vi "sub_ekf_jacob-f.vi"(10 "ud":T1, 11 "xEst":T1) -> (3 "jF":T1)   [LabVIEW 2019]
uses:
  <vilib>/Analysis/Matrix/Datatypes/RealMatrix.ctl
  Ctrl/cmd_common.ctl
  <vilib>/Analysis/Matrix/NI_Matrix.lvlib
panel:
  # "Jacobian of Motion Model\n\n    motion model\n    x_{t+1} = x_t+v*dt*cos(yaw)\n    y_{t+1} = y_t+v*dt*sin(yaw)\n    yaw_{t+1} = yaw_t+omega*dt\n    v_{t+1} = v{t}\n    so\n    dx/dyaw = -v*dt*sin(yaw)\n    dx/dv = dt*cos(yaw)\n    dy/dyaw = v*dt*cos(yaw)\n    dy/dv = dt*sin(yaw)\n    \"\"\""
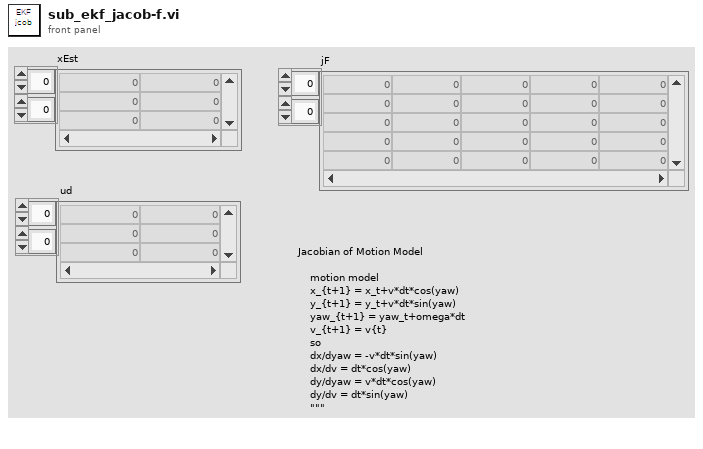
[diagram p1: front panel]
types:
  T1 = typedef "NI_Matrix.lvlib/RealMatrix.ctl" = dbl[][]
  T2 = typedef "cmd_common.ctl" = enum16{"read", "write"}
  T3 = cluster{"Q":T1, "R":T1, "input Noise":T1, "GPS noise":T1, "DT":dbl}
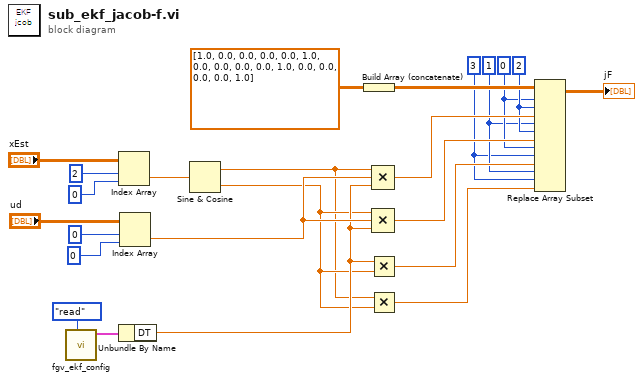
[diagram p0: block diagram]
diagram:
  w2 = 3 ("비활성화된 인덱스 (열)")
  w3 = 1 ("인덱스 (행)")
  w8 = 2 ("비활성화된 인덱스 (열)")
  w4 = 0 ("비활성화된 인덱스 (행)")
  n1 = call "fgv_ekf_config.vi"("cmd"=cmd_common."read") -> ("set var out"=w17:T3)  [unwired: 10 in]
  n2 = Index Array(array="xEst", index (row)=2 ("인덱스 (행)"), index (col)=0 ("인덱스 (열)")) -> (element=w16:dbl)
  n3 = Unbundle By Name(w17) -> ("DT"=w14:dbl)
  n4 = Index Array(array="ud", index (row)=0 ("인덱스 (행)"), index (col)=0 ("인덱스 (열)")) -> (element=w15:dbl)
  n5 = Sine & Cosine(0:w16) -> (1:w12:dbl, 2:w13:dbl)
  n6 = Build Array (concatenate)(dbl[][] [[1.0, 0.0, 0.0, 0.0], [0.0, 1.0, 0.0, 0.0], [0.0, 0.0, 1.0, 0.0], [0.0, 0.0, 0.0, 1.0]]) -> (w10:T1)
  n7 = Multiply(x=w14, y=w13) -> (x*y=w6:dbl)
  n8 = Multiply(x=w12, y=w13) -> (x*y=w5:dbl)
  n9 = Compound Arithmetic op=MULTIPLY(w12, w15, w14) -> (w9:dbl)
  n10 = Compound Arithmetic op=MULTIPLY(w13, w15, w14) -> (w7:dbl)
  n11 = Replace Array Subset(array=w10, new element #1=w9, index (row) #1=w4, index (col) #1=w8, new element #2=w7, index (row) #2=w3, index (col) #2=w8, new element #3=w6, index (row) #3=w4, index (col) #3=w2, new element #4=w5, index (row) #4=w3, index (col) #4=w2) -> (→"jF":T1)
